vi "FTW-CodeGen-GetGrowInfo.vi"(0 "State In":T2 {"Width" format="%dpx"}, 5 "XRef":refnum<vi>) -> (1 "Spacing Between Terminals":i32=8 format="%d pixels", 2 "Timing Terminal Height":i32=8 format="%d pixels", 3 "Timing Terminals":i32[](array[numeric]) format="%d pixels", 4 "Grow Info":T1, 6 "Current Height":i32=8 format="%d pixels", 8 "Width":i32=8 format="%d pixels", 10 "Terminal Height":i32=8 format="%d pixels", 13 "Bottom Banner Height":i32=8 format="%d pixels", 14 "Total Top Banner Height":i32=8 format="%d pixels")   [LabVIEW 2015, in "FTW-Dataflow-Burrow.xnode"]
uses:
  FTW-Dataflow-Burrow.xnode
  FTW-CodeGen-State.ctl
panel:
  # "Inputs"
  # "Outputs"
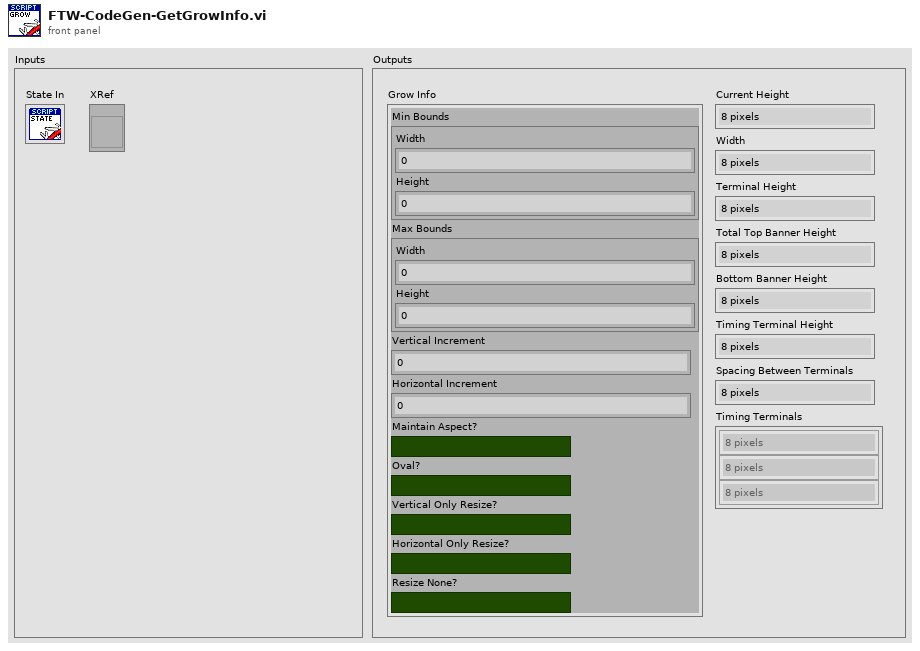
[diagram p1: front panel]
types:
  T1 = cluster{"Min Bounds":cluster{"Width":i32, "Height":i32}, "Max Bounds":cluster{"Width":i32, "Height":i32}, "Vertical Increment":i32, "Horizontal Increment":i32, "Maintain Aspect?":bool, "Oval?":bool, "Vertical Only Resize?":bool, "Horizontal Only Resize?":bool, "Resize None?":bool}
  T2 = typedef "FTW-Dataflow-Burrow.xnode/FTW-CodeGen-State.ctl" = cluster{"InputTerminals":cluster{"Wired?":bool, "ID":string, "DataName":string, "DataColor":u32, "Type":variant}[], "EnableTiming?":bool, "Width":i32}
  T3 = cluster{"Wired?":bool, "ID":string, "DataName":string, "DataColor":u32, "Type":variant}[]
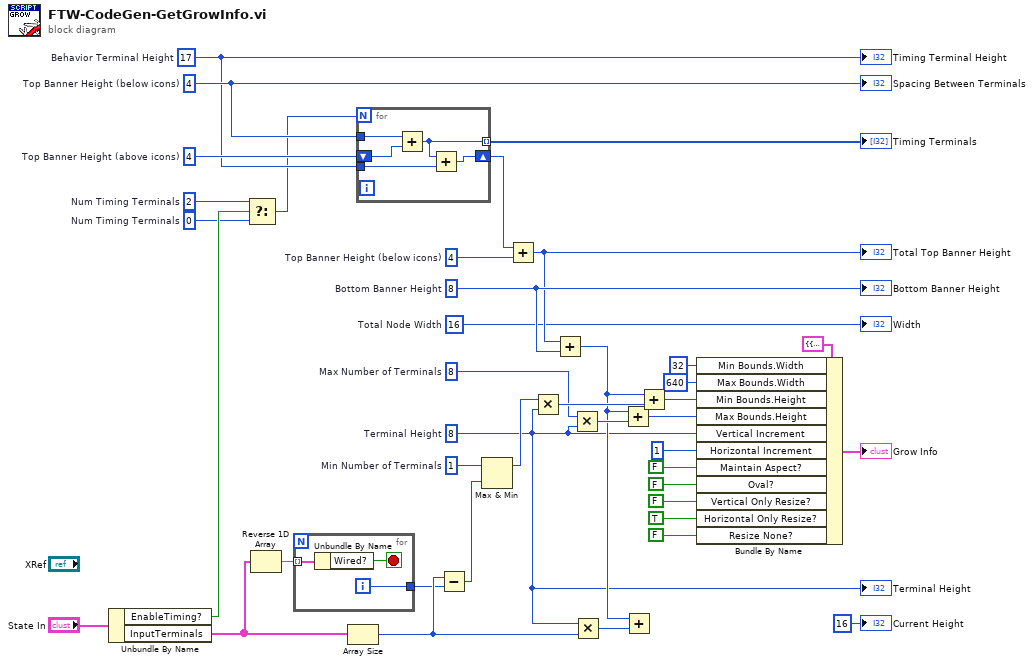
[diagram p0: block diagram]
diagram:
  w9 = 0  # Num Timing Terminals
  w11 = 2  # Num Timing Terminals
  w14 = 4  # Top Banner Height (below icons)
  w17 = 4  # Top Banner Height (below icons)
  w13 = 17  # Behavior Terminal Height
  w6 = 8  # Terminal Height
  w28 = 8  # Max Number of Terminals
  w24 = 8  # Bottom Banner Height
  w16 = 4  # Top Banner Height (above icons)
  w23 = 1  # Min Number of Terminals
  w5 = 16  # Total Node Width
  n1 = Unbundle By Name("State In") -> ("EnableTiming?"=w12:bool, "InputTerminals"=w8:T3)
  n2 = Select(t=w11, s=w12, f=w9) -> (s? t:f=w10:i32)
  n3 = Reverse 1D Array(array=w8) -> (reversed array=w21:T3)
  n4 = for {
    tunnel: w21 -> [w43] mode=indexing
    tunnel: [w42] -> w19
    i -> [w42]
    stop <- w41 stop-if-true
    n5 = Unbundle By Name(w43) -> ("Wired?"=w41:bool)
  }
  n6 = Array Size(array=w8) -> (size(s)=w20:i32)
  n7 = for {
    N: w10 -> [_]
    shift-right: [w47] -> w15
    shift-left: w16 -> [w48]
    tunnel: w13 -> [w46]
    tunnel: [w45] -> w4 mode=indexing
    tunnel: w14 -> [w44]
    n8 = Add(x=w44, y=w48) -> (x+y=w45:i32)
    n9 = Add(x=w45, y=w46) -> (x+y=w47:i32)
  }
  "Timing Terminals" <- w4
  n10 = Subtract(x=w20, y=w19) -> (x-y=w18:i32)
  n11 = Max & Min(x=w23, y=w18) -> (max(x,y)=w22:i32)  [unwired: 1 out]
  n12 = Add(x=w15, y=w17) -> (x+y=w7:i32)
  "Total Top Banner Height" <- w7
  n13 = Multiply(x=w22, y=w6) -> (x*y=w30:i32)
  n14 = Add(x=w7, y=w24) -> (x+y=w25:i32)
  n15 = Multiply(x=w28, y=w6) -> (x*y=w29:i32)
  n16 = Multiply(x=w6, y=w20) -> (x*y=w26:i32)
  n17 = Add(x=w25, y=w29) -> (x+y=w31:i32)
  n18 = Add(x=w25, y=w26) -> ()  [unwired: 1 out]
  n19 = Add(x=w25, y=w30) -> (x+y=w32:i32)
  n20 = Bundle By Name(cluster=T1 {"Min Bounds"={"Width"=0, "Height"=0}, "Max Bounds"={"Width"=0, "Height"=0}, "Vertical Increment"=0, "Horizontal Increment"=0, "Maintain Aspect?"=FALSE, "Oval?"=FALSE, "Vertical Only Resize?"=FALSE, "Horizontal Only Resize?"=FALSE, "Resize None?"=FALSE} ("Grow Info"), "Min Bounds.Width"=32, "Max Bounds.Width"=640 ("Min Bounds.Width"), "Min Bounds.Height"=w32, "Max Bounds.Height"=w31, "Vertical Increment"=w6, "Horizontal Increment"=1, "Maintain Aspect?"=FALSE, "Oval?"=FALSE, "Vertical Only Resize?"=FALSE, "Horizontal Only Resize?"=TRUE, "Resize None?"=FALSE) -> (→"Grow Info":T1)
  "Terminal Height" <- w6
  "Width" <- w5
  "Current Height" <- 16 ("Current Height")
  "Bottom Banner Height" <- w24
  "Timing Terminal Height" <- w13
  "Spacing Between Terminals" <- w14
